vi "Handle GET.vi"(8 "error in (no error)":errorcluster, 10 "parameter":string, 11 "Instrument.Framework-Template in":refnum<class "Instrument.Framework-Template.lvclass">) -> (0 "error out":errorcluster, 2 "data out":variant, 3 "Instrument.Framework-Template out":refnum<class "Instrument.Framework-Template.lvclass">)   [LabVIEW 2019, in "Instrument.Framework-Template.lvclass"]
uses:
  Instrument.Framework-Template.lvclass
  Instrument Types/SCPI/Instrument.SCPI.lvclass
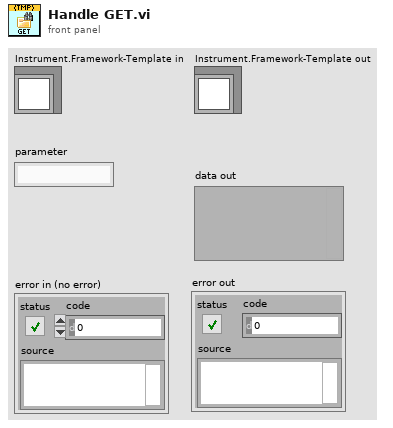
[diagram p1: front panel]
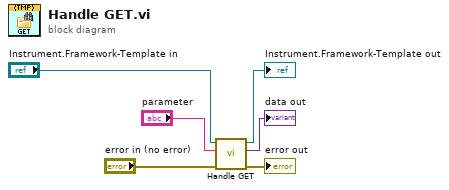
[diagram p0: block diagram]
diagram:
  n1 = call-parent "Handle GET.vi"("error in (no error)"="error in (no error)", "parameter"="parameter", "Instrument in"="Instrument.Framework-Template in") -> ("error out"=→"error out":errorcluster, "data out"=→"data out":variant, "Instrument out"=→"Instrument.Framework-Template out":refnum<class "Instrument.Framework-Template.lvclass">)  [unwired: 6 in]
